vi "amca.vi"() -> ()   [LabVIEW 2015]
uses:
  <vilib>/Enthought/Python Integration Toolkit/api/Console Visibility.ctl
  CamHandle.vi
  <vilib>/Enthought/Python Integration Toolkit/Python Integration Toolkit.lvlib
panel:
  in  "Path":path=path "C:/Users/immuser/Documents/Faster-RCNN-TensorFlow-Python3.5-master/demo_camera.py"
  in  "ADC Gain":u32=3
  out "ADC Speed (Khz)":u32=100000
  in  "Fast ADC":bool
  in  "X Start":u32=1 min=1 step=1
  in  "Y Bin":u32=2 min=1 step=1
  in  "X End":u32=2048 min=1 max=10000 step=1
  in  "X Bin":u32=2 min=1 step=1
  in  "Y Start":u32=1 min=1 step=1
  in  "Y End":u32=2048 min=1 max=10000 step=1
  in  "Temperature":dbl=37.0 format="%.2f"
  in  "Exposure":dbl=0.1 min=0.0 step=0.001 format="%.3f"
  in  "stop":bool
  in  "Store":bool
  out "error out":errorcluster={"status"=TRUE, "code"=5021, "source"="ImagePutU16Array"}
  in  "error in (no error)":errorcluster
  # "ExCoolSnapCircBufROI:\nThis example allows a single ROI\nto be programmed up. It then runs\nin sync (focus) mode displaying \nthe ROI data as it comes in.\nNote: this example requires the \ncamera support circular buffers.\nThis example also shows how to \nsetup the cascade to run in over-\nlapped mode and how to set the\non-chip multiplication gain and how\nto set the readout port."
  # "NOTICE\n\nTHIS VI USES A GLOBAL CAMERA HANDLE\n\nTHE VI EXOPENGLOBALCAM.VI MUST BE\nRUN AT THE START OF THE WORK SESSION.\nTHE CAMERA WILL REMAIN OPENED.\n\nTHE VI EXCLOSEGLOBALCAM.VI MUST\nBE RUN BEFORE LEAVING LABVIEW."
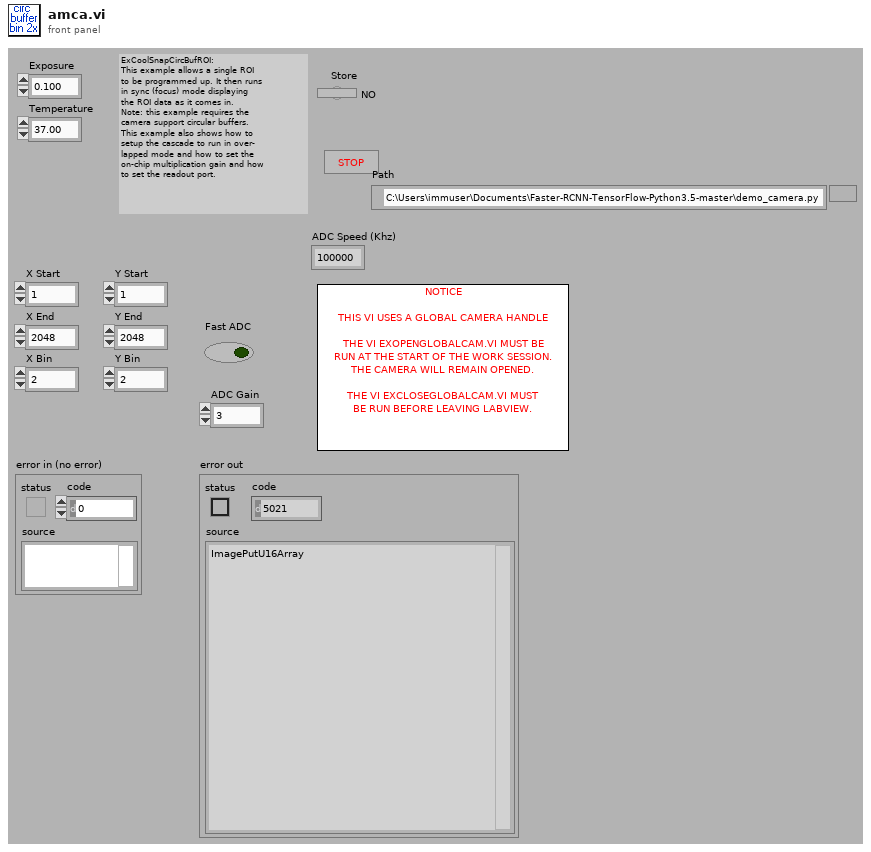
[diagram p1: front panel]
types:
  T1 = typedef "Python Integration Toolkit.lvlib/Console Visibility.ctl" = enum16{"Show Console", "Show Console While Running", "Hide Console"}
  T2 = cluster{"X Start":u32, "X End":u32, "X Bin":u32, "Y Start":u32, "Y End":u32, "Y Bin":u32}
  T3 = cluster{"acquire focus mode":u32, "Exposure":dbl, "Number of Images":u32, "Software accumulation":u32}
  T4 = typedef "Python Integration Toolkit.lvlib/Session ID.ctl" = u64
  T5 = cluster{"Camera Handle":u32, "File Handle":u32, "Display Handle":u32, "Image Handle":u32}
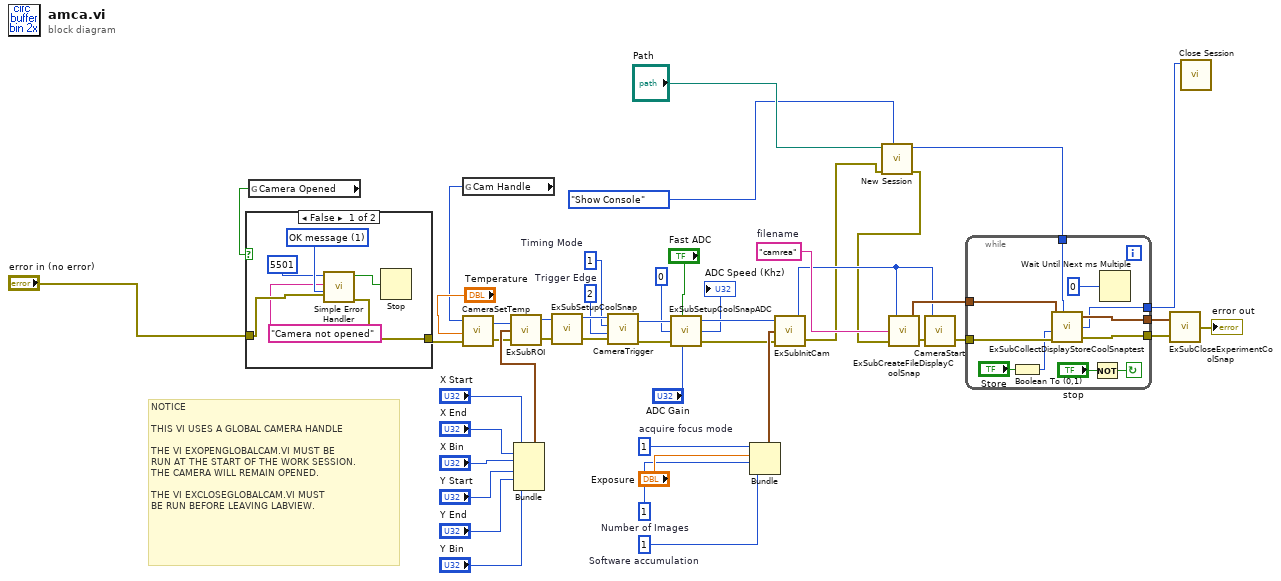
[diagram p0: block diagram]
diagram:
  w33 = u32 1  # Timing Mode
  w34 = u32 2  # Trigger Edge
  w37 = u32 1  # acquire focus mode
  w36 = u32 1  # Number of Images
  w35 = u32 1  # Software accumulation
  w45 = "camrea"  # filename
  # "NOTICE\n\nTHIS VI USES A GLOBAL CAMERA HANDLE\n\nTHE VI EXOPENGLOBALCAM.VI MUST BE\nRUN AT THE START OF THE WORK SESSION.\nTHE CAMERA WILL REMAIN OPENED.\n\nTHE VI EXCLOSEGLOBALCAM.VI MUST\nBE RUN BEFORE LEAVING LABVIEW."
  n1 = global read "CamHandle.vi" "Camera Opened"() -> (w8:bool)
  n2 = case shown="False" w8 {
    tunnel: "error in (no error)" -> [w52 w54]
    tunnel: [w51 w54] -> w9
    frame False {
      w53 = u16 1 items=["no dialog", "OK message", "continue or stop message"] ("type of dialog (OK msg:1)")
      n3 = call <vilib>:"Simple Error Handler.vi"("error code (no error:0)"=5501, "error source (\" \")"="Camera not opened", "type of dialog (OK msg:1)"=w53, "error in (no error)"=w52) -> ("error?"=w49:bool, "error out"=w51:errorcluster)  [unwired: 1 in, 3 out]
      n4 = Stop(stop? (T)=w49) -> ()
    }
    frame True {
    }
  }
  n5 = global read "CamHandle.vi" "Cam Handle"() -> (w7:u32)
  n6 = call <userlib>:"CameraSetTemp.vi"("error in (no error)"=w9, "Temperature"="Temperature", "Camera Handle"=w7) -> ("error out"=w23:errorcluster, "Camera Handle"=w22:u32)
  n7 = Bundle("X Start"="X Start", "X End"="X End", "X Bin"="X Bin", "Y Start"="Y Start", "Y End"="Y End", "Y Bin"="Y Bin") -> (w25:T2)  [unwired: 1 in]
  n8 = call "ExSubROI.vi"("error in (no error)"=w23, "ROI"=w25, "Camera Handle"=w22) -> ("error out"=w20:errorcluster, "Camera Handle"=w24:u32)
  n9 = call "ExSubSetupCoolSnap.vi"("error in (no error)"=w20, "Camera Handle"=w24) -> ("error out"=w19:errorcluster, "Camera Handle"=w40:u32)
  n10 = call <userlib>:"CameraTrigger.vi"("error in"=w19, "Trigger Edge"=w34, "Timing Mode"=w33, "Camera Handle"=w40) -> ("error out"=w17:errorcluster, "Camera Handle"=w18:u32)
  n11 = call "ExSubSetupCoolSnapADC.vi"("Camera Handle"=w18, "Fast ADC"="Fast ADC", "ReadOut Port"=0, "error in (no error)"=w17, "ADC Gain"="ADC Gain") -> ("Camera Handle"=w15:u32, "ADC Speed (Khz)"=→"ADC Speed (Khz)":u32, "error out"=w16:errorcluster)
  n12 = Bundle("acquire focus mode"=w37, "Exposure"="Exposure", "Number of Images"=w36, "Software accumulation"=w35) -> (w46:T3)  [unwired: 1 in]
  n13 = call "ExSubInitCam.vi"("error in (no error)"=w16, "Camera Information"=w46, "Camera Handle"=w15) -> ("error out"=w3:errorcluster, "Camera Handle"=w32:u32)
  n14 = call <vilib>:"New Session.vi"("Console Visibility"=Console_Visibility."Show Console", "error in (no error)"=w3, "Path to Python Module (.py File)"="Path") -> ("error out"=w2:errorcluster, "Session ID out"=w4:T4)  [unwired: 7 in]
  n15 = call "ExSubCreateFileDisplayCoolSnap.vi"("error in (no error)"=w2, "File and Display Name"=w45, "Camera Handle"=w32) -> ("error out"=w38:errorcluster, "Handles Out"=w44:T5)
  n16 = call <userlib>:"CameraStart.vi"("error in"=w38, "Camera Handle"=w32) -> ("error out"=w39:errorcluster)  [unwired: 1 out]
  n17 = while {
    tunnel: w44 -> [w64]
    tunnel: w39 -> [w63]
    tunnel: [w61] -> w42
    tunnel: [w62] -> w43
    tunnel: w4 -> [w56]
    tunnel: [w55] -> w1
    stop <- w59 continue-if-true
    n18 = Boolean To (0,1)(Boolean="Store") -> (0, 1=w57:i16)
    n19 = call "ExSubCollectDisplayStoreCoolSnaptest.vi"("Handle Cluster"=w64, "session ID"=w56, "Store flag"=w57, "error in (no error)"=w63) -> ("Handle Cluster Out"=w62:T5, "got frame"=w55:u32, "error out"=w61:errorcluster)  [unwired: 2 in]
    n20 = Not(x="stop") -> (.not. x?=w59:bool)
    n21 = Wait Until Next ms Multiple(millisecond multiple=u32 0) -> ()  [unwired: 1 out]
  }
  n22 = call "ExSubCloseExperimentCoolSnap.vi"("error in (no error)"=w42, "Handles In"=w43) -> ("error out"=→"error out":errorcluster)
  n23 = call <vilib>:"Close Session.vi"("Session ID"=w1) -> ()  [unwired: 10 in, 1 out]
